vi "sendOutputData.vi"(8 "error in (no error)":errorcluster, 11 "Model in":refnum<class "Model.lvclass">) -> (0 "error out":errorcluster, 3 "Model out":refnum<class "Model.lvclass">)   [LabVIEW 2015, in "Model.lvclass"]
uses:
  Model.lvclass
  Typedefs/OutputData.ctl
  Model.lvclass/Model.ctl
  UserEvents/UserEvents.lvclass/UserEvents.ctl
  <userlib>/Common/ILC/ILC/ILC.lvclass/ILC.ctl
  ApplicationElements/Log/TestDataLog/TestDataLog.lvclass/TestDataLog.ctl
  <userlib>/Common/ILC/ILC/ILC.lvclass
  Typedefs/M1M3SSSTypedefs.lvlib
  UserEvents/UserEvents.lvclass
  ApplicationElements/Log/TestDataLog/TestDataLog.lvclass
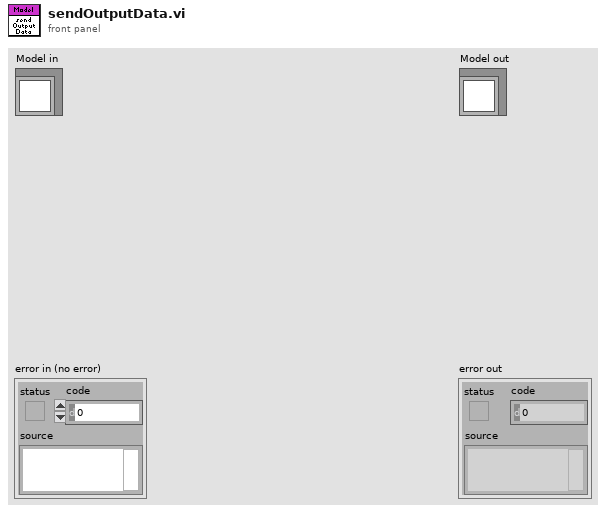
[diagram p1: front panel]
types:
  T1 = typedef "M1M3SSSTypedefs.lvlib/OutputData.ctl" = cluster{"Ramp Output":u16}
  T2 = typedef "M1M3SSSTypedefs.lvlib/PubDataEvents.ctl" = cluster{"State":refnum<user-event>, "ErrorCode":refnum<user-event>, "OutputData":refnum<user-event>, "InputData":refnum<user-event>, "ControllerData":refnum<user-event>, "TestStatus":refnum<user-event>, "LogPath":refnum<user-event>, "StiffnessData":refnum<user-event>}
  T3 = typedef "ILCCommon.lvlib/ILCTypedefs.lvlib/OutputData.ctl" = cluster{"Step & Direction":i16, "Blower RPM":u8, "PWM (SSR)":u8, "Ch1":u16, "Ch2":u16, "Ch3":u16, "Ch4":u16}
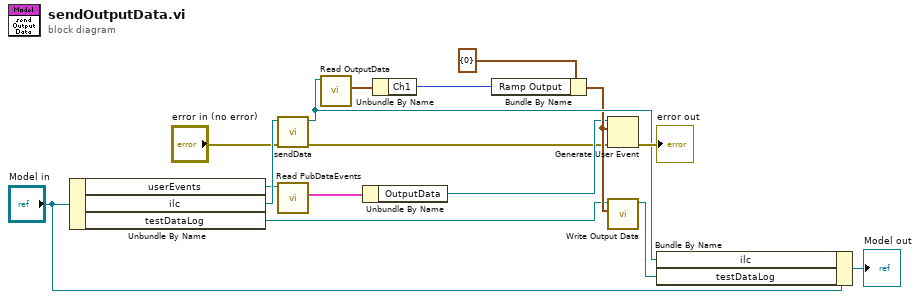
[diagram p0: block diagram]
diagram:
  n1 = Unbundle By Name("Model in") -> ("userEvents"=w2:refnum<class "UserEvents.lvclass">, "ilc"=w13:refnum<class "ILC.lvclass">, "testDataLog"=w6:refnum<class "TestDataLog.lvclass">)
  n2 = call <userlib>:"sendData.vi"("error in (no error)"="error in (no error)", "ILC in"=w13) -> ("error out"=w1:errorcluster, "ILC out"=w11:refnum<class "ILC.lvclass">)  [unwired: 8 in]
  n3 = call "Read PubDataEvents.vi"("UserEvents in"=w2) -> ("PubDataEvents"=w4:T2)  [unwired: 9 in, 1 out]
  n4 = call <userlib>:"Read OutputData.vi"("ILC in"=w11) -> ("OutputData"=w9:T3)  [unwired: 9 in, 1 out]
  n5 = Unbundle By Name(w4) -> ("OutputData"=w3:refnum<user-event>)
  n6 = Unbundle By Name(w9) -> ("Ch1"=w8:u16)
  n7 = Bundle By Name(cluster=T1 {"Ramp Output"=0} ("event data"), "Ramp Output"=w8) -> (w7:T1)
  n8 = Generate User Event(user event=w3, event data cluster=w7, error in=w1) -> (error out=→"error out":errorcluster)  [unwired: 1 in, 1 out]
  n9 = call "Write Output Data.vi"("Output Data"=w7, "Logger in"=w6) -> ("Logger out"=w5:refnum<class "TestDataLog.lvclass">)  [unwired: 9 in]
  n10 = Bundle By Name(cluster="Model in", "ilc"=w11, "testDataLog"=w5) -> (→"Model out":refnum<class "Model.lvclass">)
